vi "ParseInputStr.vi"(11 "String":string) -> (2 "Command":string[](array[string]), 3 "Data":cluster{string, string, string}[](array[cluster]))   [LabVIEW 2017]
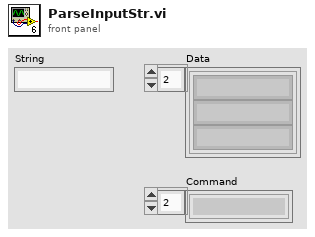
[diagram p1: front panel]
types:
  T1 = cluster{"String":string, "String":string, "String":string}
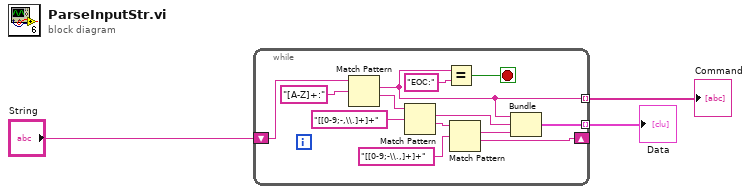
[diagram p0: block diagram]
diagram:
  n1 = while {
    shift-right: [w8] -> _
    shift-left: "String" -> [w14]
    tunnel: [w7] -> w2 mode=indexing
    tunnel: [w4] -> w3 mode=indexing
    stop <- w15 stop-if-true
    n2 = Match Pattern(string=w14, regular expression="[A-Z]+:") -> (match substring=w7:string, after substring=w12:string)  [unwired: 1 in, 2 out]
    n3 = Match Pattern(string=w12, regular expression="[[0-9;-,\\.]+]+") -> (match substring=w6:string, after substring=w9:string)  [unwired: 1 in, 2 out]
    n4 = Equal?(x=w7, y="EOC:") -> (x = y?=w15:bool)
    n5 = Match Pattern(string=w9, regular expression="[[0-9;-\\.,]+]+") -> (match substring=w5:string, after substring=w8:string)  [unwired: 1 in, 2 out]
    n6 = Bundle("String"=w7, "String"=w6, "String"=w5) -> (w4:T1)  [unwired: 1 in]
  }
  "Data" <- w3
  "Command" <- w2
